vi "Serialize - Text.vi"(8 "error in":errorcluster, 11 "M data in":refnum<class "M data.lvclass">) -> (0 "error out":errorcluster, 2 "Serialized Text":string, 3 "M data out":refnum<class "M data.lvclass">)   [LabVIEW 2014, in "Alicat Lib.lvlib" / "M data.lvclass"]
uses:
  M data.lvclass
  M data.lvclass/M data.ctl
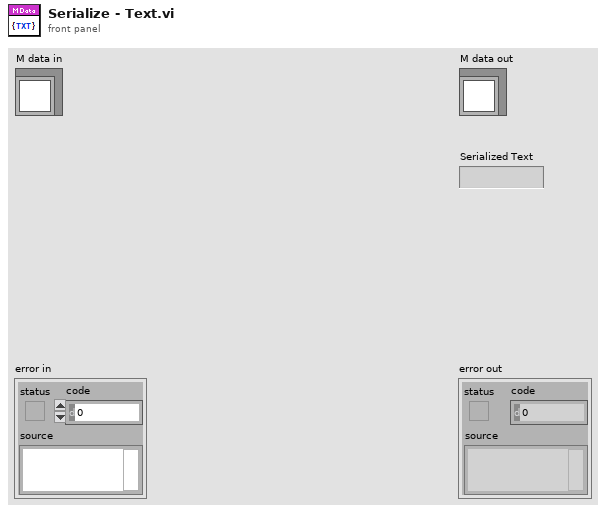
[diagram p1: front panel]
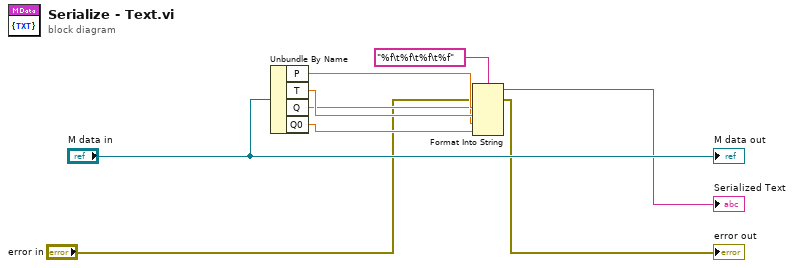
[diagram p0: block diagram]
diagram:
  n1 = Unbundle By Name("M data in") -> ("P"=w7:sgl, "T"=w6:sgl, "Q"=w5:sgl, "Q0"=w4:sgl)
  n2 = Format Into String(format string="%f\t%f\t%f\t%f", error in="error in", w7, w6, w5, w4) -> (resulting string=→"Serialized Text":string, error out=→"error out":errorcluster)  [unwired: 1 in]
  "M data out" <- "M data in"
